vi "Change in Custom Action Definition.vi"(8 "error in (no error)":errorcluster, 9 "Custom Action":T1, 10 "Selected Custom Action File Name":string, 11 "Bundle Builder in":refnum<class "Bundle Builder.lvclass">) -> (0 "error out":errorcluster, 3 "Bundle Builder out":refnum<class "Bundle Builder.lvclass">)   [LabVIEW 2020, in "Bundle Builder.lvclass"]
uses:
  Bundle Builder.lvclass
  Typedef/Custom Action Definition.ctl
  Bundle Builder.lvclass/Bundle Builder.ctl
  52107b19-8a4d-43d0-8707-c8fd6ef986f9.vi
  <vilib>/Comparison/Equal/Equal Functor/Equal Functor.lvclass
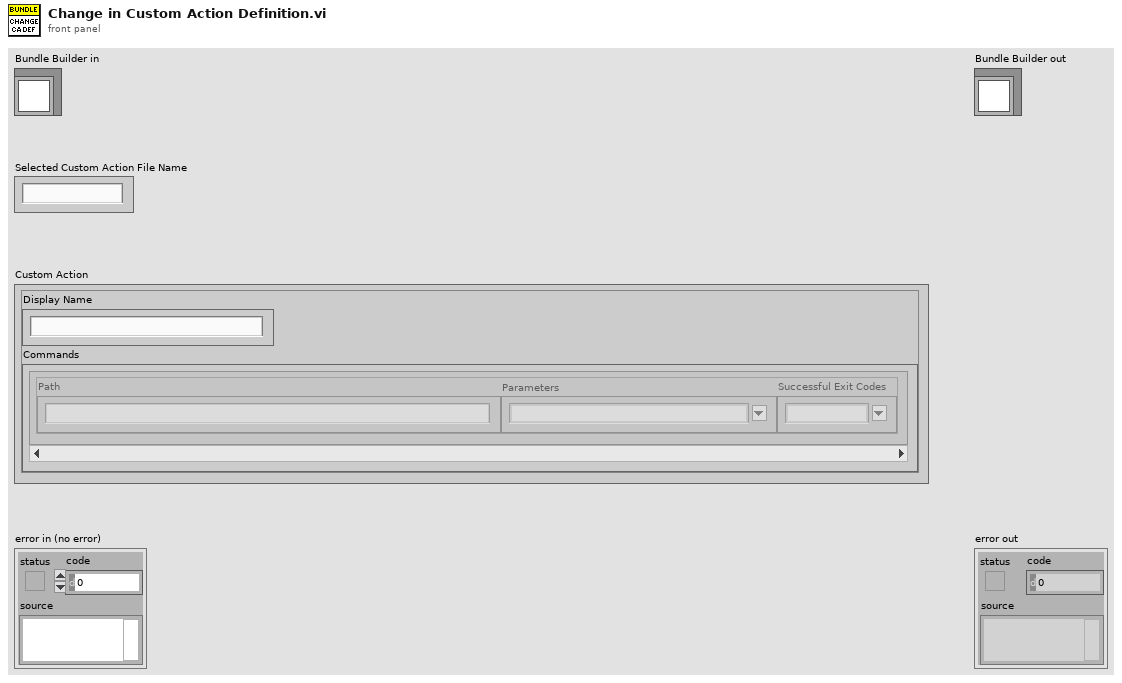
[diagram p1: front panel]
types:
  T1 = typedef "Custom Action Definition.ctl" = cluster{"Display Name":string, "Commands":cluster{"Path":string, "Parameters":string, "Successful Exit Codes":string}[]}
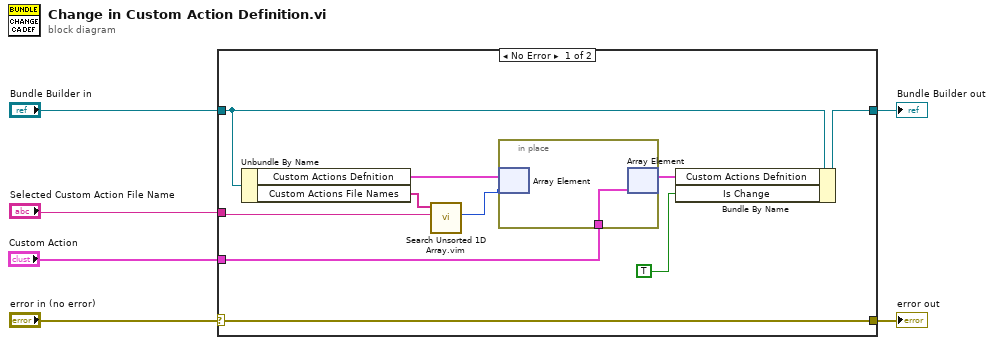
[diagram p0: block diagram]
diagram:
  n1 = case shown="No Error" "error in (no error)" {
    selector: "error in (no error)" -> [w16 w19]
    tunnel: [w16 w19] -> w5
    tunnel: [w15 w18] -> w3
    tunnel: "Bundle Builder in" -> [w14 w18]
    tunnel: "Selected Custom Action File Name" -> [w12 _]
    tunnel: "Custom Action" -> [w9 _]
    frame No Error {
      n2 = Unbundle By Name(w14) -> ("Custom Actions Defnition"=w11:T1[], "Custom Actions File Names"=w13:string[])
      n3 = call "Search Unsorted 1D Array.vim"("element"=w12, "unsorted 1D array"=w13) -> ("index of element"=w10:i32)  [unwired: 9 in]
      n4 = in-place "In Place Element Structure" {
        in-place-border: w9 -> [w17]
        n5 = in-place-array #1(w11, w10) -> ()  [unwired: 1 out]
        n6 = in-place-array #1(w17) -> (w8:T1[])  [unwired: 1 out]
      }
      n7 = Bundle By Name(cluster=w14, "Custom Actions Defnition"=w8, "Is Change"=TRUE) -> (w15:refnum<class "Bundle Builder.lvclass">)
    }
    frame Error {
    }
  }
  "error out" <- w5
  "Bundle Builder out" <- w3
